vi "BASE-Main.vi"() -> ()   [LabVIEW 2017]
uses:
  55ed0eea-cd20-493f-8468-85b8c1a0a0c0.vi
panel:
  out "Status Number":i32
  out "Status":i32(ring)=1 items=["Stopped"=1, "StartPending"=2, "StopPending"=3, "Running"=4, "ContinuePending"=5, "PausePending"=6, "Paused"=7]
  in  "RECIPE":bool
  out "error out":errorcluster
  in  "Logout":bool
  in  "Stop":bool
  in  "Create Login":bool
  in  "Parameters":bool
  in  "Start":bool
  out "Time":string
  out "Date":string
  in  "Login":bool
  # "Press Machine"
types:
  T1 = enum8{"Enabled", "Disabled", "Disabled and Grayed Out"}
  T2 = enum32{"invalid app kind", "Development System", "Run Time System", "Student Edition", "Embedded LabVIEW", "Evaluation", "Custom"}
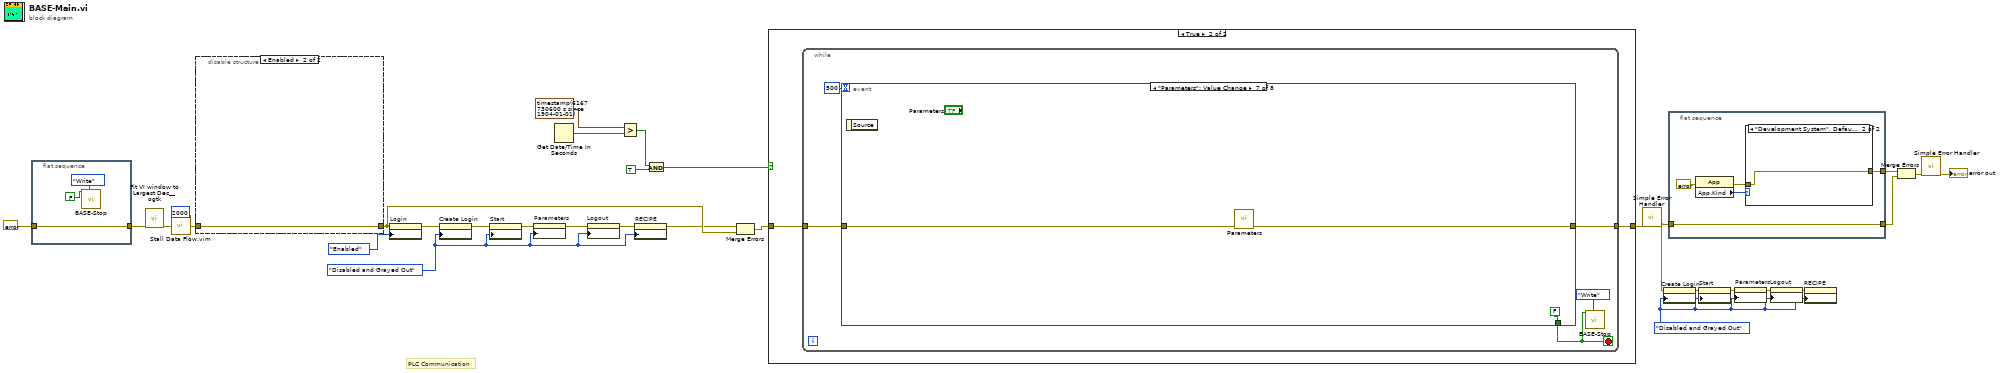
[diagram p0: block diagram]
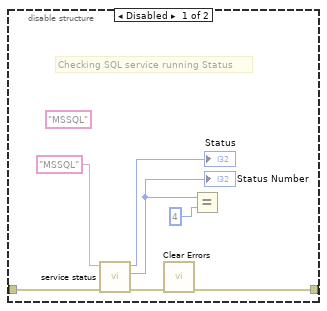
[diagram p2: hidden frame]
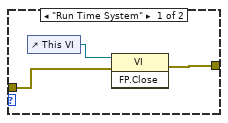
[diagram p3: hidden frame]
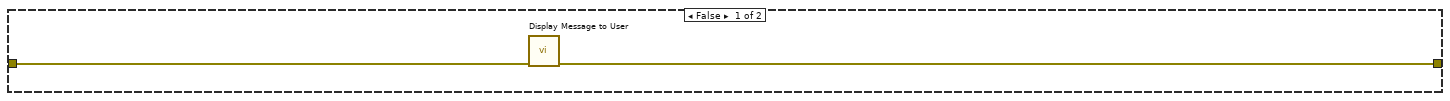
[diagram p4: hidden frame]
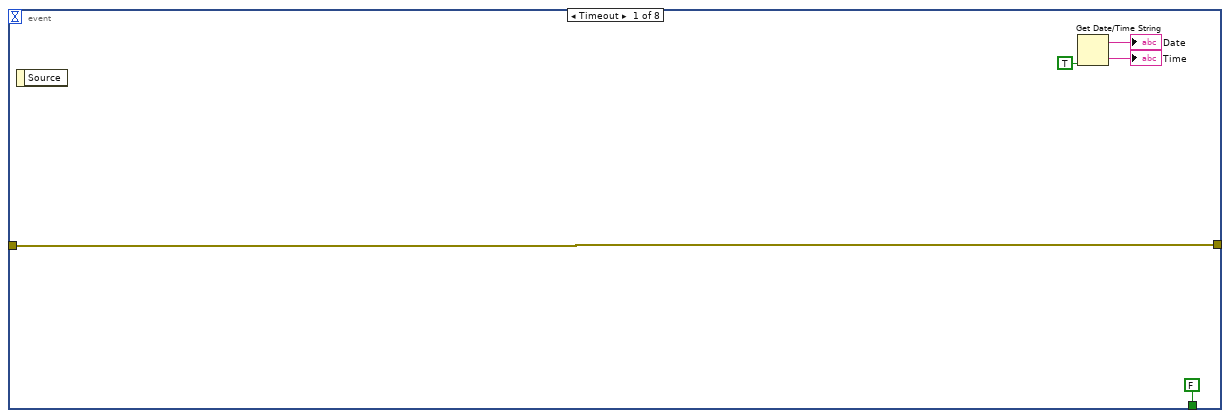
[diagram p5: hidden frame]
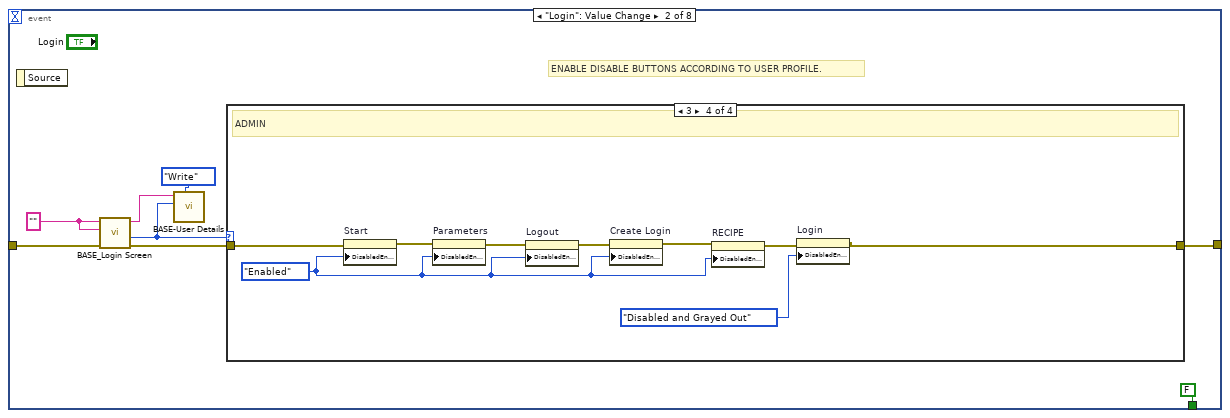
[diagram p6: hidden frame]
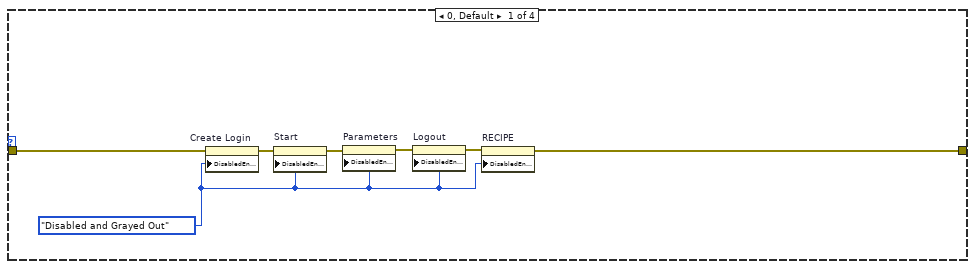
[diagram p7: hidden frame]
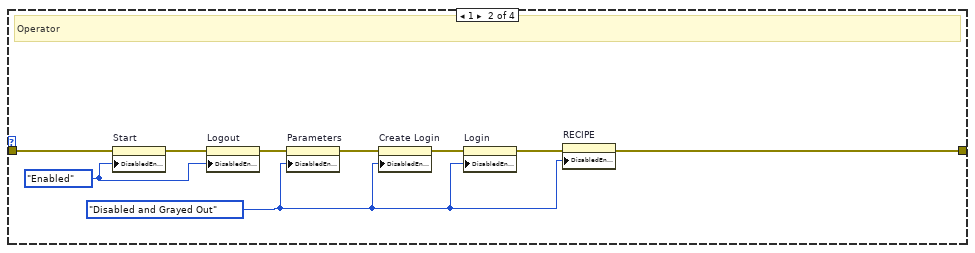
[diagram p8: hidden frame]
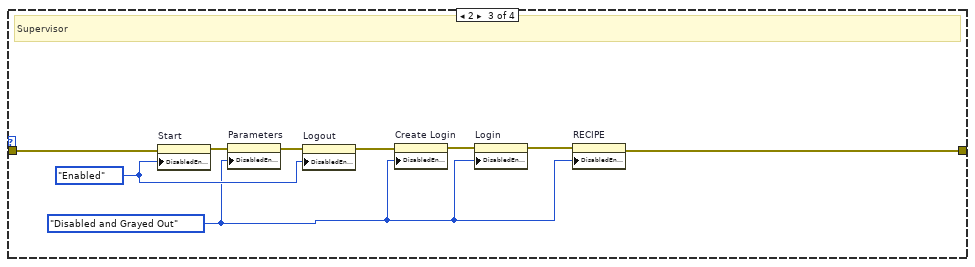
[diagram p9: hidden frame]
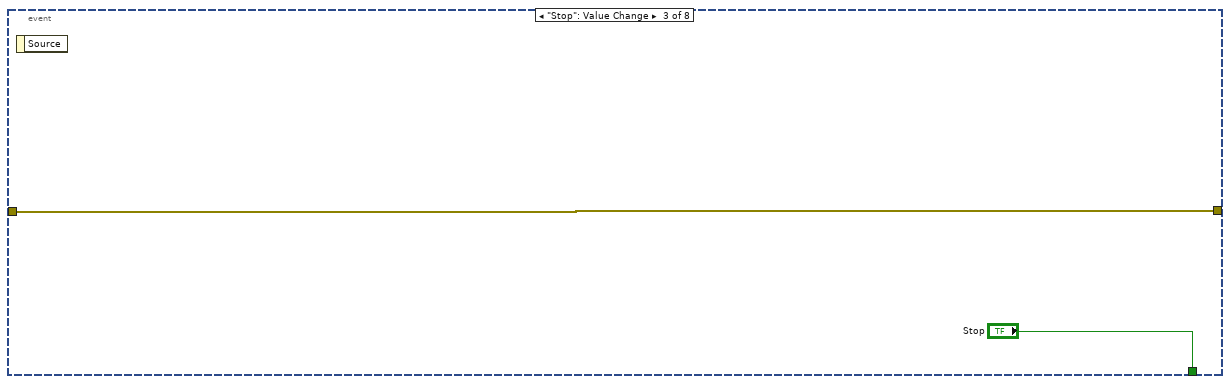
[diagram p10: hidden frame]
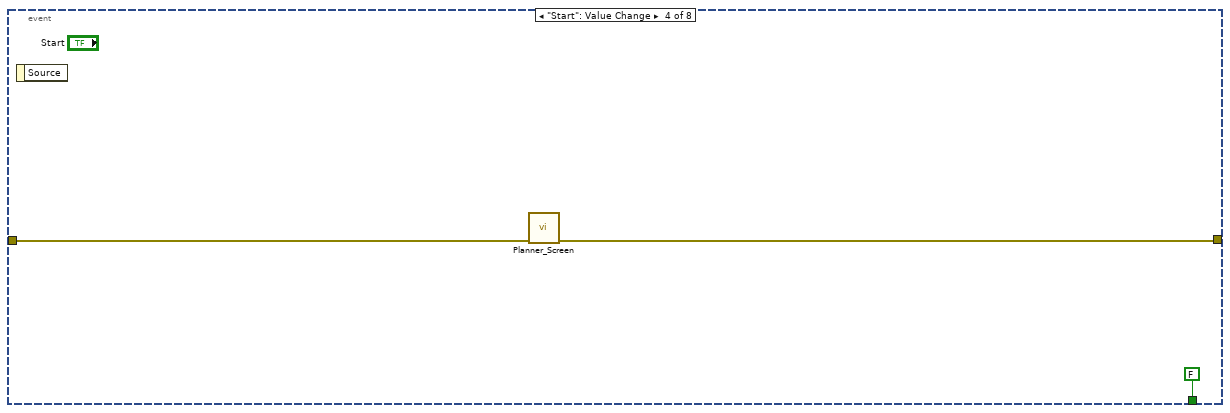
[diagram p11: hidden frame]
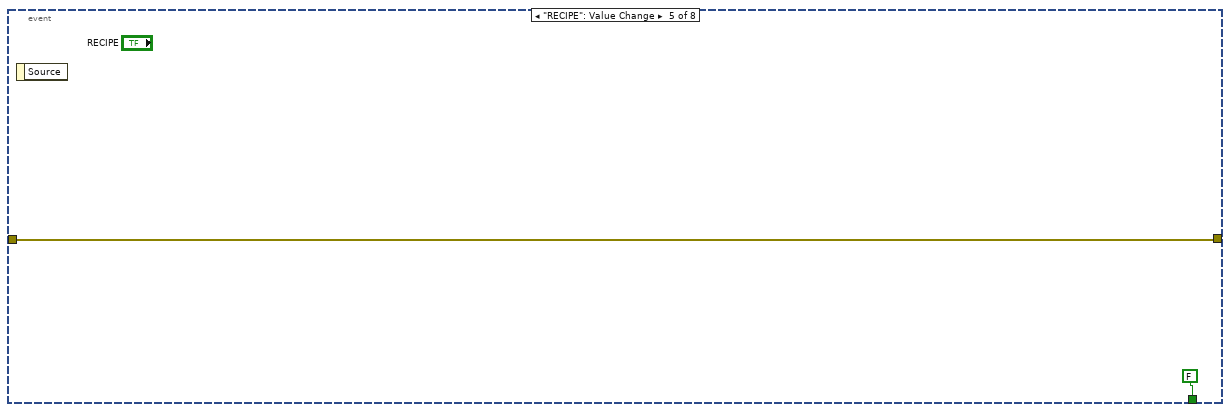
[diagram p12: hidden frame]
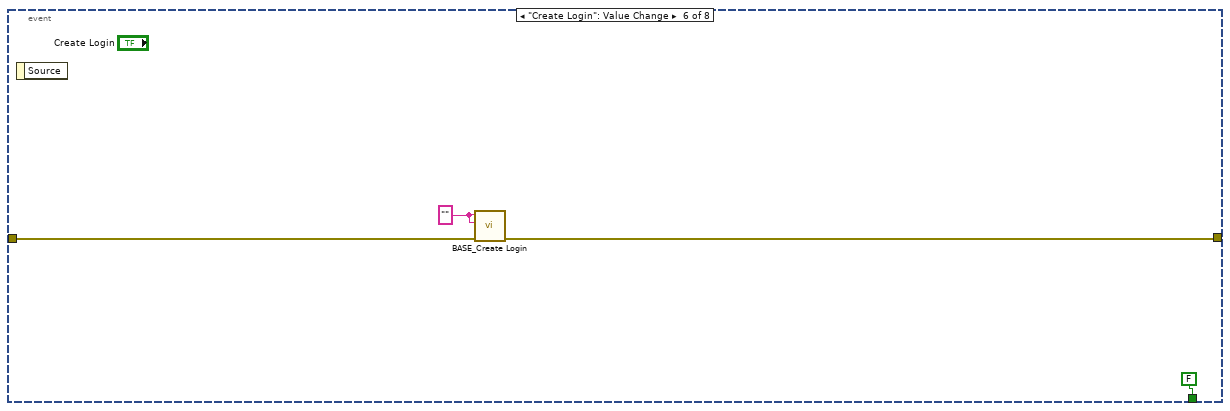
[diagram p13: hidden frame]
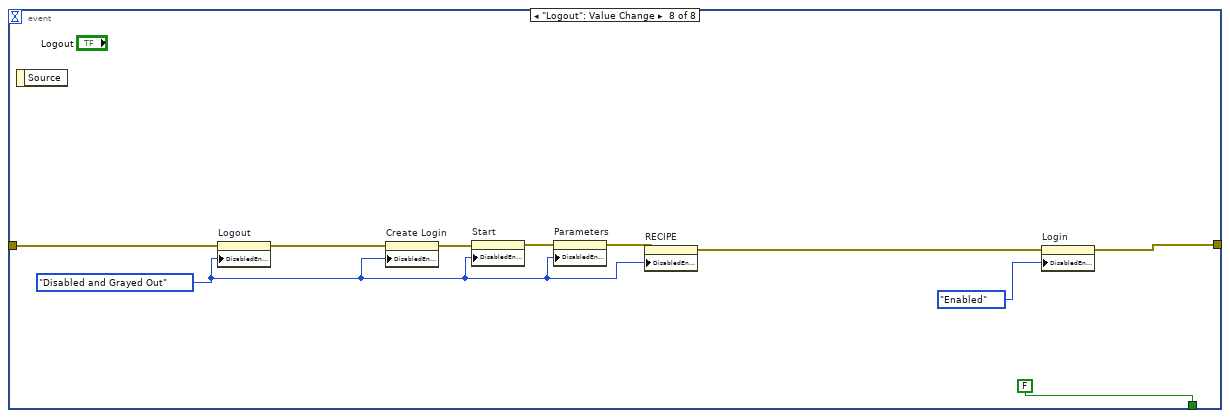
[diagram p14: hidden frame]
diagram:
  w8 = T1."Disabled and Grayed Out" ("Disabled")
  w9 = T1."Disabled and Grayed Out" ("Disabled")
  # "PLC Communication"
  n1 = flat-sequence {
    tunnel: [w34] -> w22
    tunnel: errorcluster {"status"=FALSE, "code"=0, "source"=""} ("error constant") -> [w34]
    frame #0 {
      n2 = call "BASE-Stop.vi"("Enum"=enum16{"Read", "Write"}."Write", "Stop"=FALSE) -> ()  [unwired: 9 in, 1 out]
    }
  }
  n3 = call <userlib>:"Fit VI window to Largest Dec__ogtk.vi"("error in (no error)"=w22) -> ("error out"=w14:errorcluster)  [unwired: 5 in, 1 out]
  n4 = call "Stall Data Flow.vim"("value in"=w14, "milliseconds to wait"=u32 2000) -> ("value out"=w13:errorcluster)  [unwired: 1 out]
  n5 = disable-structure shown="Enabled" {
    disable-tunnel: [w36 w42] -> w19
    disable-tunnel: w13 -> [w35 w42]
    frame Disabled {
      (unwired) "MSSQL" ("Service Name")
      # "Checking SQL service running Status"
      n6 = call "service status.vi"("error in"=w35, "Service Name"="MSSQL") -> ("error out"=w37:errorcluster, "Status Number"=w39:i32, "Status"=→"Status":i32)  [unwired: 6 in, 1 out]
      "Status Number" <- w39
      n7 = call <vilib>:"Clear Errors.vi"("error in (no error)"=w37) -> ("error out"=w36:errorcluster)  [unwired: 5 in, 1 out]
      n8 = Equal?(x=w39, y=4) -> ()  [unwired: 1 out]
    }
    frame Enabled {
    }
  }
  n9 = property on="Login" class="Bool"(error in=w19, "DisabledEnum"=T1."Enabled" ("Disabled")) -> (error out=w26:errorcluster)  [unwired: 1 in, 1 out]
  n10 = property on="Create Login" class="Bool"(error in=w26, "DisabledEnum"=w9) -> (error out=w30:errorcluster)  [unwired: 1 in, 1 out]
  n11 = property on="Start" class="Bool"(error in=w30, "DisabledEnum"=w9) -> (error out=w10:errorcluster)  [unwired: 1 in, 1 out]
  n12 = property on="Parameters" class="Bool"(error in=w10, "DisabledEnum"=w9) -> (error out=w24:errorcluster)  [unwired: 1 in, 1 out]
  n13 = Get Date/Time In Seconds() -> (seconds since 1Jan1904=w16:timestamp)
  n14 = property on="Logout" class="Bool"(error in=w24, "DisabledEnum"=w9) -> (error out=w11:errorcluster)  [unwired: 1 in, 1 out]
  n15 = Greater?(x=timestamp(6167730600 s since 1904-01-01), y=w16) -> (0:w15:bool)
  n16 = property on="RECIPE" class="Bool"(error in=w11, "DisabledEnum"=w9) -> (error out=w2:errorcluster)  [unwired: 1 in, 1 out]
  n17 = And(x=w15, y=TRUE) -> (x .and. y?=w18:bool)
  n18 = Merge Errors(w2, w19) -> (w21:errorcluster)
  n19 = case shown="True" w18 {
    tunnel: w21 -> [w44 w46]
    tunnel: [w43 w45] -> w31
    frame False {
      n20 = call "Display Message to User"("error in (no error)"=w44) -> ("error out"=w43:errorcluster)  [unwired: 9 in, 1 out]
    }
    frame True {
      n21 = while {
        tunnel: w46 -> [w50]
        tunnel: [w49] -> w45
        stop <- w47 stop-if-true
        n22 = event shown="[6] \"Parameters\": Value Change" {
          selector: _ -> [_ _ _ _ _ _ _ _]
          dyn-events: _ -> [_ _ _ _ _ _ _ _]
          timeout: 500 -> [_ _ _ _ _ _ _ _]
          tunnel: w50 -> [w54 w64 w99 w102 w104 w109 w111 w119]
          tunnel: [w54 w57 w99 w101 w104 w108 w110 w120] -> w49
          tunnel: [FALSE ("Stop") FALSE ("Stop") "Stop" FALSE ("Stop") FALSE ("Stop") FALSE ("Stop") FALSE ("Stop") FALSE ("Stop")] -> w47
          event Timeout {
            n23 = event-data() -> ()  [unwired: 1 in, 1 out]
            n24 = Get Date/Time String(want seconds? (F)=TRUE) -> (date string=→"Date":string, time string=→"Time":string)  [unwired: 2 in]
          }
          event "Login": Value Change {
            w60 = "" ("User Name")
            # "ENABLE DISABLE BUTTONS ACCORDING TO USER PROFILE."
            n25 = event-data() -> ()  [unwired: 1 in, 1 out]
            n26 = call "BASE_Login Screen.vi"("Error In"=w64, "Password"=w60, "User Name"=w60) -> ("error out"=w63:errorcluster, "Level"=w58:i32, "User Name Out"=w61:string)  [unwired: 5 in, 1 out]
            n27 = call "BASE-User Details.vi"("Enum"=enum16{"Read", "Write"}."Write", "Level In"=w58, "User Name In"=w61) -> ()  [unwired: 7 in, 2 out]
            n28 = case shown="3" w58 {
              tunnel: w63 -> [w69 w80 w89 w98]
              tunnel: [w65 w73 w82 w90] -> w57
              frame 0, Default {
                w66 = T1."Disabled and Grayed Out" ("Disabled")
                n29 = property on="Create Login" class="Bool"(error in=w69, "DisabledEnum"=w66) -> (error out=w71:errorcluster)  [unwired: 1 in, 1 out]
                n30 = property on="Start" class="Bool"(error in=w71, "DisabledEnum"=w66) -> (error out=w70:errorcluster)  [unwired: 1 in, 1 out]
                n31 = property on="Parameters" class="Bool"(error in=w70, "DisabledEnum"=w66) -> (error out=w67:errorcluster)  [unwired: 1 in, 1 out]
                n32 = property on="Logout" class="Bool"(error in=w67, "DisabledEnum"=w66) -> (error out=w68:errorcluster)  [unwired: 1 in, 1 out]
                n33 = property on="RECIPE" class="Bool"(error in=w68, "DisabledEnum"=w66) -> (error out=w65:errorcluster)  [unwired: 1 in, 1 out]
              }
              frame 1 {
                w72 = T1."Disabled and Grayed Out" ("Disabled")
                w74 = T1."Enabled" ("Disabled")
                # "Operator"
                n34 = property on="Start" class="Bool"(error in=w80, "DisabledEnum"=w74) -> (error out=w76:errorcluster)  [unwired: 1 in, 1 out]
                n35 = property on="Logout" class="Bool"(error in=w76, "DisabledEnum"=w74) -> (error out=w78:errorcluster)  [unwired: 1 in, 1 out]
                n36 = property on="Parameters" class="Bool"(error in=w78, "DisabledEnum"=w72) -> (error out=w79:errorcluster)  [unwired: 1 in, 1 out]
                n37 = property on="Create Login" class="Bool"(error in=w79, "DisabledEnum"=w72) -> (error out=w77:errorcluster)  [unwired: 1 in, 1 out]
                n38 = property on="Login" class="Bool"(error in=w77, "DisabledEnum"=w72) -> (error out=w75:errorcluster)  [unwired: 1 in, 1 out]
                n39 = property on="RECIPE" class="Bool"(error in=w75, "DisabledEnum"=w72) -> (error out=w73:errorcluster)  [unwired: 1 in, 1 out]
              }
              frame 2 {
                w81 = T1."Disabled and Grayed Out" ("Disabled")
                w83 = T1."Enabled" ("Disabled")
                # "Supervisor"
                n40 = property on="Start" class="Bool"(error in=w89, "DisabledEnum"=w83) -> (error out=w86:errorcluster)  [unwired: 1 in, 1 out]
                n41 = property on="Parameters" class="Bool"(error in=w86, "DisabledEnum"=w81) -> (error out=w88:errorcluster)  [unwired: 1 in, 1 out]
                n42 = property on="Logout" class="Bool"(error in=w88, "DisabledEnum"=w83) -> (error out=w84:errorcluster)  [unwired: 1 in, 1 out]
                n43 = property on="Create Login" class="Bool"(error in=w84, "DisabledEnum"=w81) -> (error out=w87:errorcluster)  [unwired: 1 in, 1 out]
                n44 = property on="Login" class="Bool"(error in=w87, "DisabledEnum"=w81) -> (error out=w85:errorcluster)  [unwired: 1 in, 1 out]
                n45 = property on="RECIPE" class="Bool"(error in=w85, "DisabledEnum"=w81) -> (error out=w82:errorcluster)  [unwired: 1 in, 1 out]
              }
              frame 3 {
                w91 = T1."Enabled" ("Disabled")
                # "ADMIN"
                n46 = property on="Start" class="Bool"(error in=w98, "DisabledEnum"=w91) -> (error out=w93:errorcluster)  [unwired: 1 in, 1 out]
                n47 = property on="Parameters" class="Bool"(error in=w93, "DisabledEnum"=w91) -> (error out=w97:errorcluster)  [unwired: 1 in, 1 out]
                n48 = property on="Logout" class="Bool"(error in=w97, "DisabledEnum"=w91) -> (error out=w96:errorcluster)  [unwired: 1 in, 1 out]
                n49 = property on="Create Login" class="Bool"(error in=w96, "DisabledEnum"=w91) -> (error out=w95:errorcluster)  [unwired: 1 in, 1 out]
                n50 = property on="RECIPE" class="Bool"(error in=w95, "DisabledEnum"=w91) -> (error out=w94:errorcluster)  [unwired: 1 in, 1 out]
                n51 = property on="Login" class="Bool"(error in=w94, "DisabledEnum"=T1."Disabled and Grayed Out" ("Disabled")) -> (error out=w90:errorcluster)  [unwired: 1 in, 1 out]
              }
            }
          }
          event "Stop": Value Change {
            n52 = event-data() -> ()  [unwired: 1 in, 1 out]
          }
          event "Start": Value Change {
            n53 = event-data() -> ()  [unwired: 1 in, 1 out]
            n54 = call "Planner_Screen.vi"("error in (no error)"=w102) -> ("error out"=w101:errorcluster)  [unwired: 10 in]
          }
          event "RECIPE": Value Change {
            n55 = event-data() -> ()  [unwired: 1 in, 1 out]
          }
          event "Create Login": Value Change {
            w107 = "" ("User Name")
            n56 = event-data() -> ()  [unwired: 1 in, 1 out]
            n57 = call "BASE_Create Login.vi"("Error In"=w109, "Password"=w107, "User Name"=w107) -> ("error out"=w108:errorcluster)  [unwired: 6 in]
          }
          event "Parameters": Value Change {
            n58 = event-data() -> ()  [unwired: 1 in, 1 out]
            n59 = call "Parameters.vi"("error in (no error)"=w111) -> ("error out"=w110:errorcluster)  [unwired: 10 in]
          }
          event "Logout": Value Change {
            w114 = T1."Disabled and Grayed Out" ("Disabled")
            n60 = event-data() -> ()  [unwired: 1 in, 1 out]
            n61 = property on="Logout" class="Bool"(error in=w119, "DisabledEnum"=w114) -> (error out=w115:errorcluster)  [unwired: 1 in, 1 out]
            n62 = property on="Create Login" class="Bool"(error in=w115, "DisabledEnum"=w114) -> (error out=w122:errorcluster)  [unwired: 1 in, 1 out]
            n63 = property on="Start" class="Bool"(error in=w122, "DisabledEnum"=w114) -> (error out=w121:errorcluster)  [unwired: 1 in, 1 out]
            n64 = property on="Parameters" class="Bool"(error in=w121, "DisabledEnum"=w114) -> (error out=w116:errorcluster)  [unwired: 1 in, 1 out]
            n65 = property on="RECIPE" class="Bool"(error in=w116, "DisabledEnum"=w114) -> (error out=w113:errorcluster)  [unwired: 1 in, 1 out]
            n66 = property on="Login" class="Bool"(error in=w113, "DisabledEnum"=T1."Enabled" ("Disabled")) -> (error out=w120:errorcluster)  [unwired: 1 in, 1 out]
          }
        }
        n67 = call "BASE-Stop.vi"("Enum"=enum16{"Read", "Write"}."Write", "Stop"=w47) -> ()  [unwired: 9 in, 1 out]
      }
    }
  }
  n68 = call <vilib>:"Simple Error Handler.vi"("error in (no error)"=w31) -> ("error out"=w3:errorcluster)  [unwired: 4 in, 4 out]
  n69 = property on="Create Login" class="Bool"(error in=w3, "DisabledEnum"=w8) -> (error out=w4:errorcluster)  [unwired: 1 in, 1 out]
  n70 = flat-sequence {
    tunnel: [w124] -> w29
    tunnel: [w123] -> w27
    tunnel: w3 -> [w123]
    frame #0 {
      n71 = property class="App"(error in=errorcluster {"status"=FALSE, "code"=0, "source"=""} ("error in (no error)")) -> (error out=w126:errorcluster, "App.Kind"=w127:T2)  [unwired: 1 in, 1 out]
      n72 = case shown="\"Development System\", Default" w127 {
        tunnel: w126 -> [w129 w131]
        tunnel: [w128 w131] -> w124
        frame "Run Time System" {
          n73 = control-ref of="This VI"() -> (w130:refnum<vi>)
          n74 = invoke class="VI" method="FP.Close"(reference=w130, error in=w129) -> (error out=w128:errorcluster)  [unwired: 1 in, 2 out]
        }
        frame "Development System", Default {
        }
      }
    }
  }
  n75 = property on="Start" class="Bool"(error in=w4, "DisabledEnum"=w8) -> (error out=w7:errorcluster)  [unwired: 1 in, 1 out]
  n76 = property on="Parameters" class="Bool"(error in=w7, "DisabledEnum"=w8) -> (error out=w5:errorcluster)  [unwired: 1 in, 1 out]
  n77 = property on="Logout" class="Bool"(error in=w5, "DisabledEnum"=w8) -> (error out=w6:errorcluster)  [unwired: 1 in, 1 out]
  n78 = property on="RECIPE" class="Bool"(error in=w6, "DisabledEnum"=w8) -> ()  [unwired: 1 in, 2 out]
  n79 = Merge Errors(w29, w27) -> (w28:errorcluster)
  n80 = call <vilib>:"Simple Error Handler.vi"("error in (no error)"=w28) -> ("error out"=→"error out":errorcluster)  [unwired: 4 in, 4 out]
